vi "Close ColorProcessorSDK.vi"(8 "error in (no error)":errorcluster, 11 "ColorProcessorSDK reference":refnum<k24>) -> (0 "error out":errorcluster)   [LabVIEW 2020]
uses:
  C:/GEECS/Developers Version/builds/Device builds/ThorlabsCsCamera/Thorlabs.TSI.ColorProcessor.dll
  Thorlabs.TSI.ColorProcessor.dll
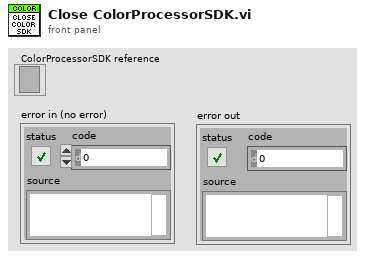
[diagram p1: front panel]
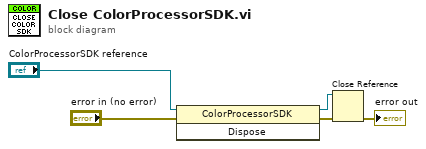
[diagram p0: block diagram]
diagram:
  n1 = invoke class="ColorProcessorSDK" method="Dispose"(reference="ColorProcessorSDK reference", error in="error in (no error)") -> (reference out=w2:refnum<k24>, error out=w3:errorcluster)  [unwired: 1 in, 1 out]
  n2 = Close Reference(reference=w2, error in (no error)=w3) -> (error out=→"error out":errorcluster)
